vi "Set Injected Value static.vi"(8 "error in (no error)":errorcluster, 10 "Value":T1, 11 "Abs_Single Float in":refnum<class "Abs_Single Float.lvclass">) -> (0 "error out":errorcluster, 3 "Abs_Single Float out":refnum<class "Abs_Single Float.lvclass">)   [LabVIEW 2021, in "Fault-Injection_SGL.lvclass"]
uses:
  Fault-Injection_SGL.lvclass
  Value Type.ctl
  Fault-Injection_SGL.lvclass/Fault-Injection_SGL.ctl
  C:/Program Files (x86)/National Instruments/LabVIEW 2021/vi.lib/TSA/Abstract Data Classes/Abs_Types/Single Float/Abs_Single Float.lvclass
  C:/Program Files (x86)/National Instruments/LabVIEW 2021/vi.lib/TSA/Abstract Data Classes/Abs_Types/Floating Point/Abs_Floating Point.lvclass
  C:/Program Files (x86)/National Instruments/LabVIEW 2021/vi.lib/TSA/Abstract Data Classes/Abs_Types/Numeric/Abs_Numeric.lvclass
  C:/Program Files (x86)/National Instruments/LabVIEW 2021/vi.lib/TSA/Abstract Data Classes/Abs_Types/Value/Abs_Value.lvclass
  C:/Program Files (x86)/National Instruments/LabVIEW 2021/vi.lib/TSA/Abstract Data Classes/Abs_Types/Type/Abs_Type.lvclass
  C:/Users/Tim/Documents/GitHub/Omni-Bus/Source/Fault-Injection Bus/Support/Interfaces/SGL/Fault-Injection_SGL_Type.lvclass
  C:/Users/Tim/Documents/GitHub/Omni-Bus/Source/Fault-Injection Bus/Support/Interfaces/Type/Fault-Injection_Type.lvclass
  C:/Users/Tim/Documents/GitHub/Omni-Bus/Source/Fault-Injection Bus/Support/Value Type/SGL/Fault-Injection_SGL.lvclass
  <vilib>/TSA/Abstract Data Classes/Abs_Types/Single Float/Abs_Single Float.lvclass
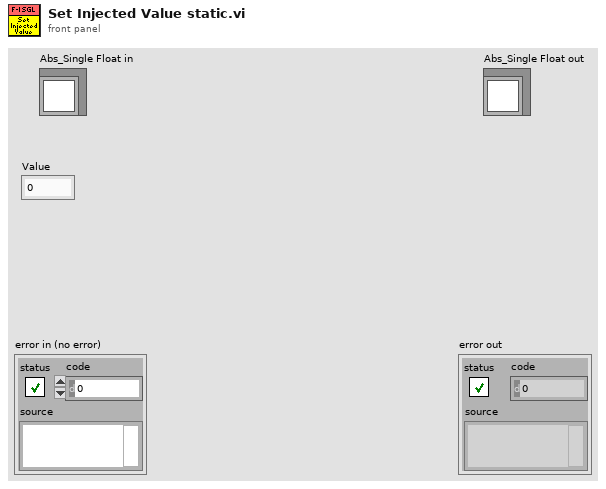
[diagram p1: front panel]
types:
  T1 = typedef "Fault-Injection_SGL.lvclass/Value Type.ctl" = sgl
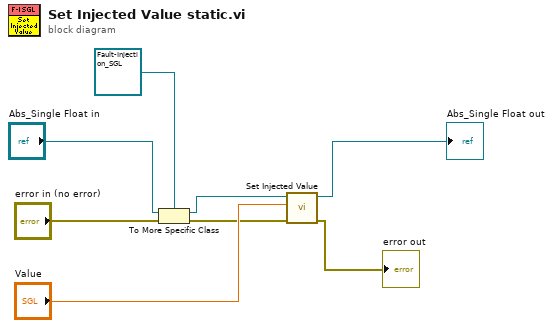
[diagram p0: block diagram]
diagram:
  n1 = To More Specific Class(target class=refnum<class "Fault-Injection_SGL.lvclass"> refnum ("Fault-Injection_Boolean in"), reference="Abs_Single Float in", error in="error in (no error)") -> (specific class reference=w1:refnum<class "Fault-Injection_SGL.lvclass">, error out=w5:errorcluster)
  n2 = call-dynamic "Set Injected Value.vi"("error in (no error)"=w5, "Value"="Value", "Fault-Injection_Boolean in"=w1) -> ("error out"=→"error out":errorcluster, "Fault-Injection_Boolean out"=→"Abs_Single Float out":refnum<class "Fault-Injection_SGL.lvclass">)  [unwired: 7 in]
